vi "Receive Message.vi"(8 "error in (no error)":errorcluster, 10 "timeout ms (5000)":i32=1000, 11 "WebSocket Connection in":refnum<k5>) -> (0 "error out":errorcluster, 1 "data (JSON)":string, 2 "msg (string)":string, 3 "WebSocket Connection out":refnum<k5>)   [LabVIEW 2014]
uses:
  <vilib>/Intelligent Energy/WebSockets API/WebSockets/WebSockets.lvlib
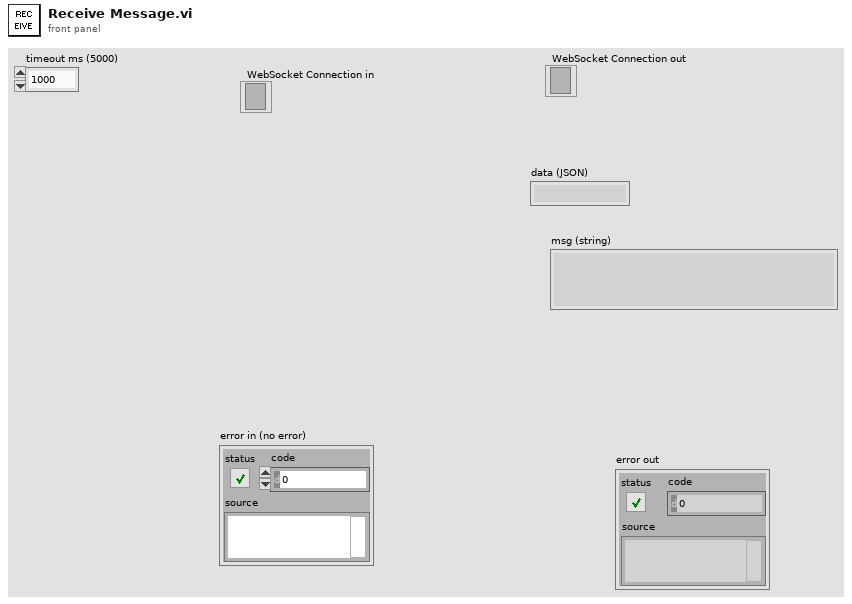
[diagram p1: front panel]
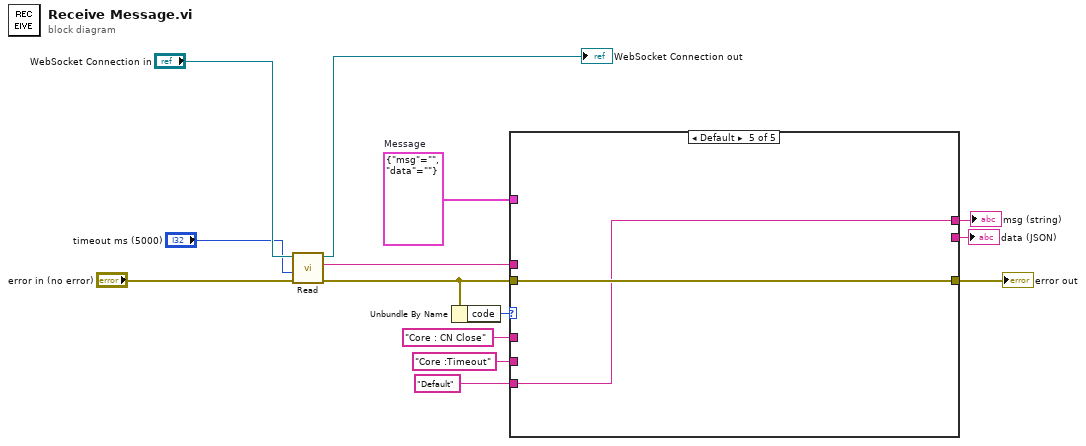
[diagram p0: block diagram]
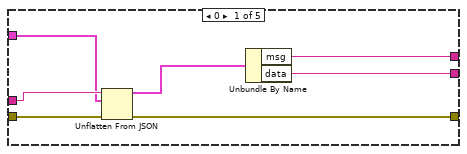
[diagram p2: hidden frame]
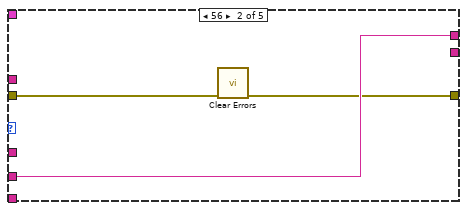
[diagram p3: hidden frame]
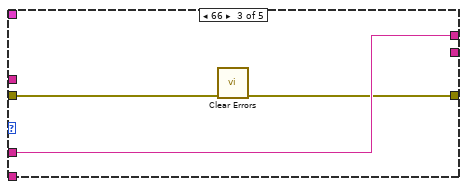
[diagram p4: hidden frame]
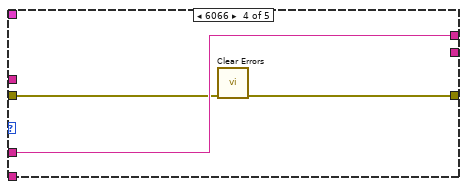
[diagram p5: hidden frame]
diagram:
  w4 = cluster{"msg":string, "data":string} {"msg"="", "data"=""}  # Message
  n1 = call <vilib>:"Read.vi"("error in (no error)"="error in (no error)", "timeout ms (5000)"="timeout ms (5000)", "WebSocket Connection in"="WebSocket Connection in") -> ("error out"=w7:errorcluster, "Data"=w5:string, "WebSocket Connection out"=→"WebSocket Connection out":refnum<k5>)  [unwired: 5 in, 1 out]
  n2 = Unbundle By Name(w7) -> ("code"=w10:i32)
  n3 = case shown="Default" w10 {
    tunnel: [w16 w23 w26 w30 w31] -> w8
    tunnel: "Core :Timeout" ("Msg") -> [_ w23 _ _ _]
    tunnel: w7 -> [w21 w24 w27 w29 w32]
    tunnel: [w20 w22 w25 w28 w32] -> w6
    tunnel: w5 -> [w19 _ _ _ _]
    tunnel: w4 -> [w18 _ _ _ _]
    tunnel: [w15 _ _ _ _] -> w3
    tunnel: "Default" ("data") -> [_ _ _ _ w31]
    tunnel: "Core : CN Close" ("msg") -> [_ _ w26 w30 _]
    frame 0 {
      n4 = Unflatten From JSON(JSON string=w19, type and defaults=w18, error in (no error)=w21) -> (value=w17:cluster{"msg":string, "data":string}, error out=w20:errorcluster)  [unwired: 4 in]
      n5 = Unbundle By Name(w17) -> ("msg"=w16:string, "data"=w15:string)
    }
    frame 56 {
      n6 = call <vilib>:"Clear Errors.vi"("error in (no error)"=w24) -> ("error out"=w22:errorcluster)  [unwired: 5 in, 1 out]
    }
    frame 66 {
      n7 = call <vilib>:"Clear Errors.vi"("error in (no error)"=w27) -> ("error out"=w25:errorcluster)  [unwired: 5 in, 1 out]
    }
    frame 6066 {
      n8 = call <vilib>:"Clear Errors.vi"("error in (no error)"=w29) -> ("error out"=w28:errorcluster)  [unwired: 5 in, 1 out]
    }
    frame Default {
    }
  }
  "error out" <- w6
  "msg (string)" <- w8
  "data (JSON)" <- w3
